vi "Register Field Value Change Events.vi"(8 "error in (no error)":errorcluster, 10 "Field Event Refnum In":refnum<event-registration>, 11 "Panel Form Controller in":refnum<class "Panel Form Controller.lvclass">) -> (0 "error out":errorcluster, 2 "Field Event Refnum Out":refnum<event-registration>, 3 "Panel Form Controller out":refnum<class "Panel Form Controller.lvclass">)   [LabVIEW 2020, in "Panel Form Controller.lvlib" / "Panel Form Controller.lvclass"]
uses:
  Panel Form Controller.lvclass
  Panel Form Controller.lvclass/Panel Form Controller.ctl
  Field.lvclass/Field.ctl
  Field.lvclass
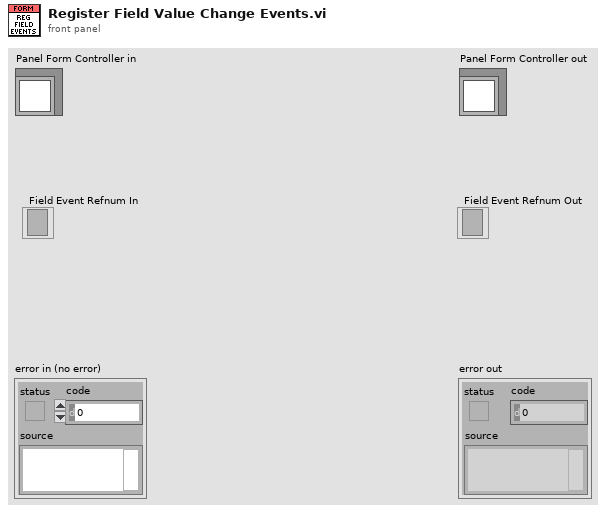
[diagram p1: front panel]
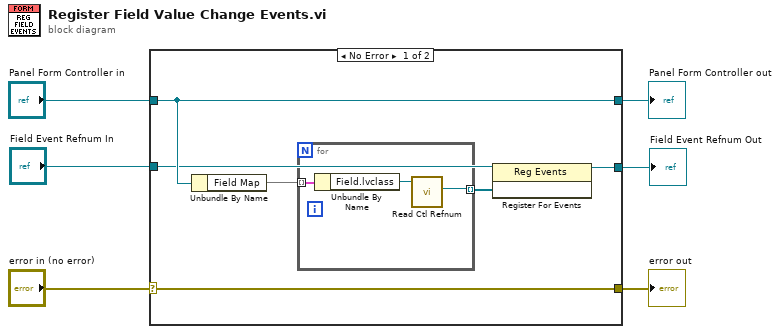
[diagram p0: block diagram]
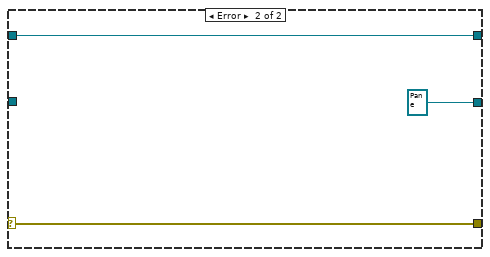
[diagram p2: hidden frame]
diagram:
  n1 = case shown="No Error" "error in (no error)" {
    selector: "error in (no error)" -> [w12 w18]
    tunnel: [w12 w18] -> w5
    tunnel: [w11 w17] -> w3
    tunnel: "Panel Form Controller in" -> [w11 w17]
    tunnel: [w8 refnum<event-registration> refnum ("field value change")] -> w2
    tunnel: "Field Event Refnum In" -> [w7 _]
    frame No Error {
      n2 = Unbundle By Name(w11) -> ("Field Map"=w10:map{string, refnum<class "Field.lvclass">})
      n3 = for {
        tunnel: w10 -> [w15] mode=indexing
        tunnel: [w13] -> w9 mode=indexing
        n4 = Unbundle By Name(w15) -> ("Field.lvclass"=w14:refnum<class "Field.lvclass">)
        n5 = call "Read Ctl Refnum.vi"("Field in"=w14) -> ("Ctl Refnum"=w13:refnum<vi>)  [unwired: 8 in, 2 out]
      }
      n6 = register-events(reference=w7, w9) -> (reference out=w8:refnum<event-registration>)  [unwired: 1 in, 1 out]
    }
    frame Error {
    }
  }
  "error out" <- w5
  "Panel Form Controller out" <- w3
  "Field Event Refnum Out" <- w2
